vi "ReceiveWaveform.vi"(8 "error in (no error)":errorcluster, 10 "Waveform":waveform(dbl), 11 "TopUI in":refnum<class "TopUI.lvclass">) -> (0 "error out":errorcluster, 3 "TopUI out":refnum<class "TopUI.lvclass">)   [LabVIEW 2020, in "TopUI.lvlib" / "TopUI.lvclass"]
uses:
  TopUI.lvclass
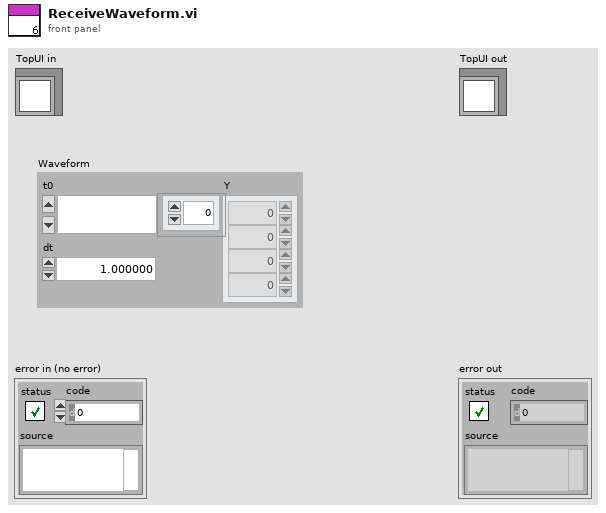
[diagram p1: front panel]
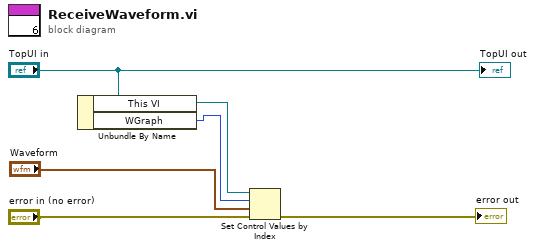
[diagram p0: block diagram]
diagram:
  n1 = Unbundle By Name("TopUI in") -> ("This VI"=w3:refnum<vi>, "WGraph"=w2:i32)
  n2 = Set Control Values by Index(0:w3, 1:w2, 2:"Waveform", 3:"error in (no error)") -> (11:→"error out":errorcluster)
  "TopUI out" <- "TopUI in"
